vi "Recall Value from TDMS.vi"(6 "Value":variant, 7 "Prefix":string, 8 "Error In":errorcluster, 9 "channel name":string, 10 "group name":string, 11 "tdms file":refnum<k34>) -> (0 "Error Out":errorcluster, 1 "channel name out":string, 2 "group name out":string, 3 "tdms file out":refnum<k34>, 4 "Value out":variant)   [LabVIEW 2016]
uses:
  <vilib>/Utility/Data Type/Type Definitions/Data Type.ctl
  <vilib>/Utility/Data Type/NI_Data Type.lvlib
panel:
  out "found":bool
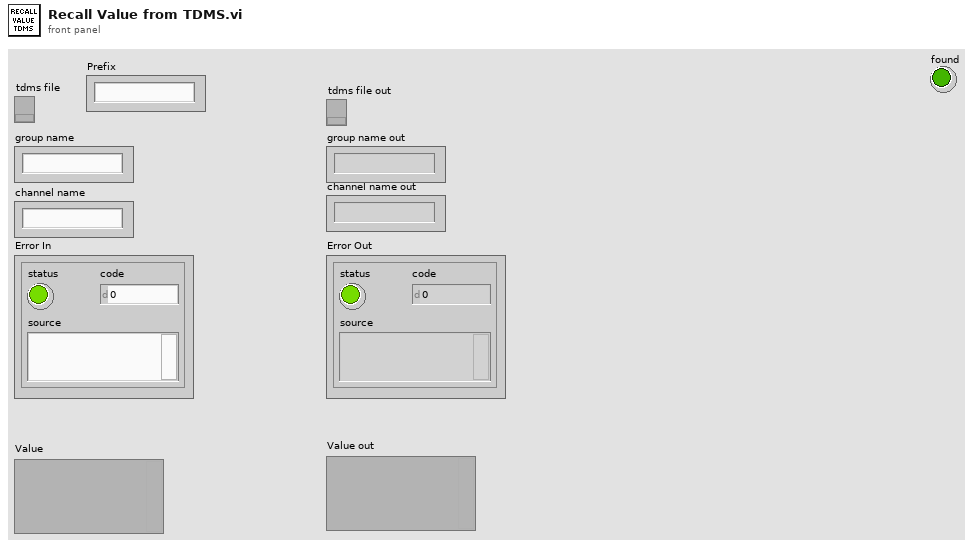
[diagram p1: front panel]
types:
  T1 = typedef "NI_Data Type.lvlib/Data Type.ctl" = enum8{"Invalid Type", "Void", "I8", "I16", "I32", "I64", "U8", "U16", "U32", "U64", "Single Float", "Double Float", "Extended Float", "Single Complex", "Double Complex", "Extended Complex", "Enum U8", "Enum U16", "Enum U32", "Enum U64", "Single Float With Unit", "Double Float With Unit", "Extended Float With Unit", "Single Complex with Unit", "Double Complex with Unit", "Extended Complex with Unit", "Boolean", "String", "Path", "Picture", "Tag", "Array", "Cluster", "Variant", "LV Variant", "Waveform", "Timestamp", "Digital Waveform", "Digital Data", "ExpressData", "Refnum", "External Data", "VI", "Poly VI", "LabVIEW Class Instance", "Fixed Point"}
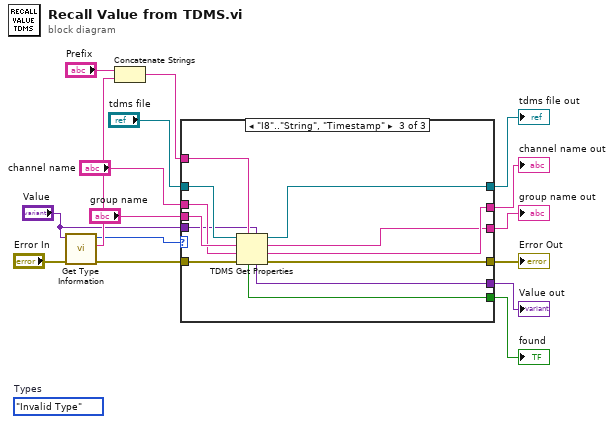
[diagram p0: block diagram]
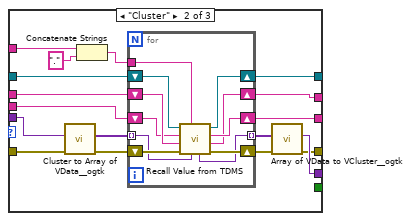
[diagram p3: hidden frame]
diagram:
  (unwired) Data_Type."Invalid Type"  # Types
  n1 = call <vilib>:"Get Type Information.vi"("error in (no error)"="Error In", "Variant"="Value") -> ("error out"=w7:errorcluster, "Name"=w9:string, "Type"=w6:T1)  [unwired: 5 in, 2 out]
  n2 = Concatenate Strings("Prefix", w9) -> (w2:string)
  n3 = case shown="\"I8\"..\"String\", \"Timestamp\"" w6 {
    tunnel: "tdms file" -> [w20 w30 w60]
    tunnel: [w20 w29 w59] -> w15
    tunnel: "group name" -> [w18 w21 w58]
    tunnel: "channel name" -> [w17 w22 w57]
    tunnel: [w17 w27 w56] -> w12
    tunnel: [w18 w28 w55] -> w11
    tunnel: w7 -> [w19 w33 w54]
    tunnel: [w19 w24 w53] -> w10
    tunnel: w2 -> [_ w32 w52]
    tunnel: "Value" -> [_ w31 w51]
    tunnel: [_ _ w50] -> w4
    tunnel: [_ w25 w49] -> w3
    frame "Invalid Type", Default {
    }
    frame "Cluster" {
      n4 = call <userlib>:"Cluster to Array of VData__ogtk.vi"("error in (no error)"=w33, "Cluster"=w31) -> ("error out"=w37:errorcluster, "Array of VData"=w36:variant[])  [unwired: 8 in]
      n5 = Concatenate Strings(w32, "." ("string")) -> (w35:string)
      n6 = for {
        shift-right: [w45] -> w23
        shift-left: w37 -> [w47]
        shift-right: [w46] -> w29
        shift-left: w30 -> [w48]
        shift-right: [w40] -> w27
        shift-left: w22 -> [w39]
        shift-right: [w41] -> w28
        shift-left: w21 -> [w38]
        tunnel: w36 -> [w44] mode=indexing
        tunnel: w35 -> [w43]
        tunnel: [w42] -> w26 mode=indexing
        n7 = call "Recall Value from TDMS.vi"("Value"=w44, "Prefix"=w43, "Error In"=w47, "channel name"=w39, "group name"=w38, "tdms file"=w48) -> ("Error Out"=w45:errorcluster, "channel name out"=w40:string, "group name out"=w41:string, "tdms file out"=w46:refnum<k34>, "Value out"=w42:variant)  [unwired: 1 in]
      }
      n8 = call <userlib>:"Array of VData to VCluster__ogtk.vi"("error in (no error)"=w23, "Array"=w26) -> ("error out"=w24:errorcluster, "VCluster"=w25:variant)  [unwired: 8 in]
    }
    frame "I8".."String", "Timestamp" {
      n9 = TDMS Get Properties(5:w51, 7:w52, 8:w54, 9:w57, 10:w58, 11:w60) -> (0:w53:errorcluster, 1:w56:string, 2:w55:string, 3:w59:refnum<k34>, 4:w49:variant, 6:w50:bool)
    }
  }
  "Error Out" <- w10
  "tdms file out" <- w15
  "channel name out" <- w12
  "group name out" <- w11
  "found" <- w4
  "Value out" <- w3
